vi "AutoPush.vi"(7 "PushMode":T1, 10 "RPM":dbl, 11 "MotorIn":dbl) -> (3 "MotorOut":dbl)   [LabVIEW 2013]
uses:
  SingleSolenoidAction.ctl
  PushMode.ctl
panel:
  in  "Increase in Power/s":dbl
  in  "Decrease Power/s":dbl
  in  "MaxAccel (rpm/s)":dbl
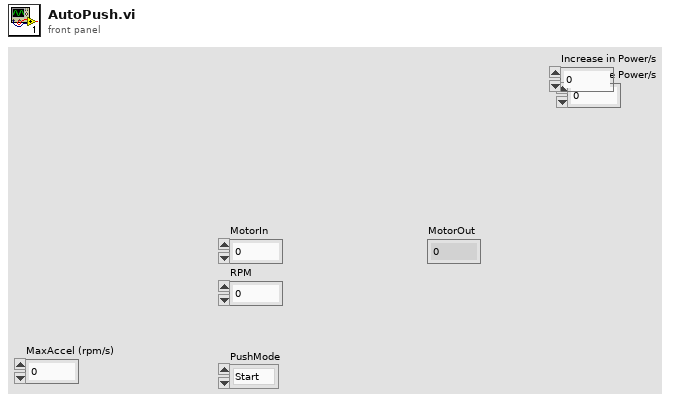
[diagram p1: front panel]
types:
  T1 = typedef "PushMode.ctl" = enum16{"Start", "Adjust", "Stop"}
  T2 = typedef "SingleSolenoidAction.ctl" = enum16{"Init", "SetState", "Disable"}
  T3 = enum16{"Power Maintain", "Power Decrease", "Power Increase"}
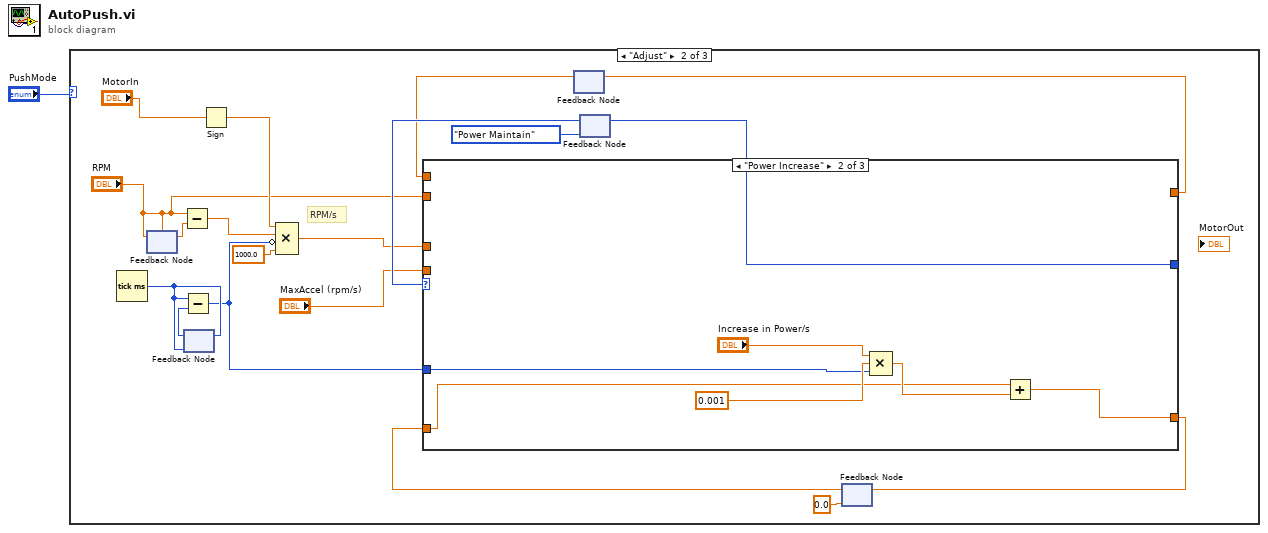
[diagram p0: block diagram]
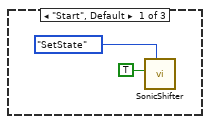
[diagram p2: hidden frame]
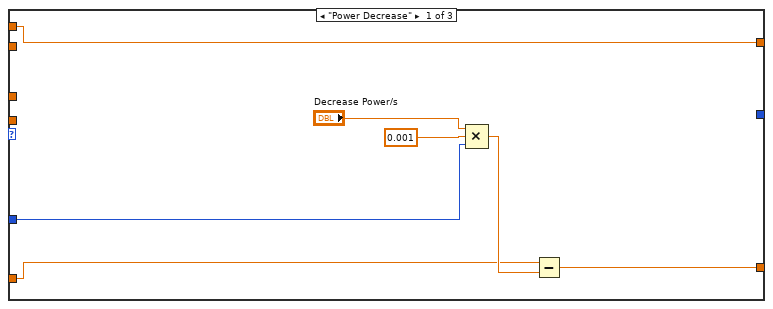
[diagram p3: hidden frame]
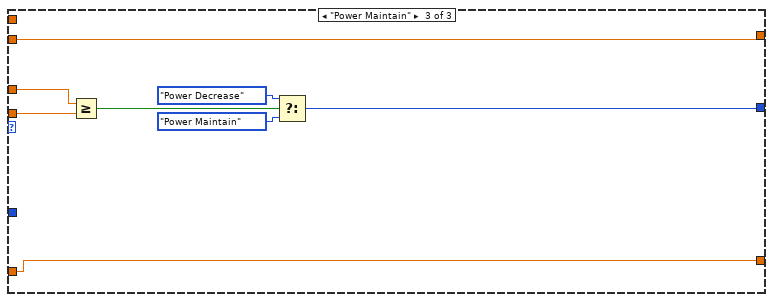
[diagram p4: hidden frame]
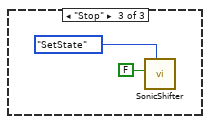
[diagram p5: hidden frame]
diagram:
  n1 = case shown="\"Adjust\"" "PushMode" {
    frame "Start", Default {
      n2 = call "SonicShifter.vi"("Action"=SingleSolenoidAction."SetState" ("Mode"), "Actuate?"=TRUE) -> ()  [unwired: 9 in, 1 out]
    }
    frame "Adjust" {
      # "RPM/s"
      n3 = Tick Count (ms)() -> (millisecond timer value=w21:u32)
      n4 = feedback #1("RPM") -> (w20:dbl)
      n5 = feedback-in #1("RPM") -> ()
      n6 = Subtract(x="RPM", y=w20) -> (x-y=w15:dbl)
      n7 = feedback #2(w21) -> (w22:u32)
      n8 = Subtract(x=w21, y=w22) -> (x-y=w9:u32)
      n9 = feedback-in #2(w21) -> ()
      n10 = Sign(1:"MotorIn") -> (0:w18:dbl)
      n11 = Compound Arithmetic op=MULTIPLY(w18, w15, invert w9, 1000.0 ("value")) -> (w8:dbl)
      n12 = feedback #3() -> (w5:dbl)  [unwired: 1 in]
      n13 = feedback #4(T3."Power Maintain" ("Enum")) -> (w16:T3)
      n14 = feedback #5(0.0) -> (w10:dbl)
      n15 = case shown="\"Power Increase\"" w16 {
        tunnel: w8 -> [_ _ w43]
        tunnel: "MaxAccel (rpm/s)" -> [_ _ w42]
        tunnel: [_ _ w38] -> w11
        tunnel: w10 -> [w24 w31 w36]
        tunnel: w9 -> [w25 w32 _]
        tunnel: "RPM" -> [_ _ w37]
        tunnel: [w29 _ w37] -> w6
        tunnel: w5 -> [w29 _ _]
        tunnel: [w23 w30 w36] -> w4
        frame "Power Decrease" {
          n16 = Compound Arithmetic op=MULTIPLY("Decrease Power/s", 0.001, w25) -> (w26:dbl)
          n17 = Subtract(x=w24, y=w26) -> (x-y=w23:dbl)
        }
        frame "Power Increase" {
          n18 = Compound Arithmetic op=MULTIPLY("Increase in Power/s", 0.001, w32) -> (w33:dbl)
          n19 = Add(x=w31, y=w33) -> (x+y=w30:dbl)
        }
        frame "Power Maintain" {
          n20 = Greater Or Equal?(x=w43, y=w42) -> (x >= y?=w41:bool)
          n21 = Select(t=T3."Power Decrease" ("Enum"), s=w41, f=T3."Power Maintain" ("Enum")) -> (s? t:f=w38:T3)
        }
      }
      n22 = feedback-in #3(w6) -> ()
      n23 = feedback-in #4(w11) -> ()
      n24 = feedback-in #5(w4) -> ()
    }
    frame "Stop" {
      n25 = call "SonicShifter.vi"("Action"=SingleSolenoidAction."SetState" ("Mode"), "Actuate?"=FALSE) -> ()  [unwired: 9 in, 1 out]
    }
  }
